vi "Facade.vi"(0 "Data In":T4, 2 "Display State In":T2, 3 "Container State":T3) -> (6 "Data Out":T4, 7 "Display State Out":T2, 8 "Action":T1)   [LabVIEW 2015, in "TTLWaterDelivery.xctl"]
uses:
  TTLWaterDelivery.xctl
  Data.ctl
  Device Classes/WaterDelivery Class/TTLWaterDelivery.lvclass
  <vilib>/_xctls/Container State.ctl
  State.ctl
  <vilib>/_xctls/Action.ctl
  Device Classes/WaterDelivery Class/TTLWaterDelivery.lvclass/TTLWaterDelivery.ctl
  Device Classes/WaterDelivery Class/Read uL_ms.vi
  Device Classes/WaterDelivery Class/Write uL_ms.vi
  <vilib>/_xctls/XControlSupport.lvlib
panel:
  in  "Calibrate":bool
  in  "Sensitivity":dbl format="%#_g ul/ms"
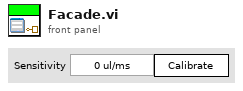
[diagram p1: front panel]
types:
  T1 = typedef "XControlSupport.lvlib/Action.ctl" = cluster{"Data Changed?":bool, "State Changed?":bool, "Action Name":string}
  T2 = typedef "TTLWaterDelivery.xctl/State.ctl" = cluster{"Cal signal":refnum<vi>}
  T3 = typedef "XControlSupport.lvlib/Container State.ctl" = cluster{"Indicator?":bool, "Run Mode?":bool, " Refnum":refnum<vi>}
  T4 = typedef "TTLWaterDelivery.xctl/Data.ctl" = refnum<class "TTLWaterDelivery.lvclass">
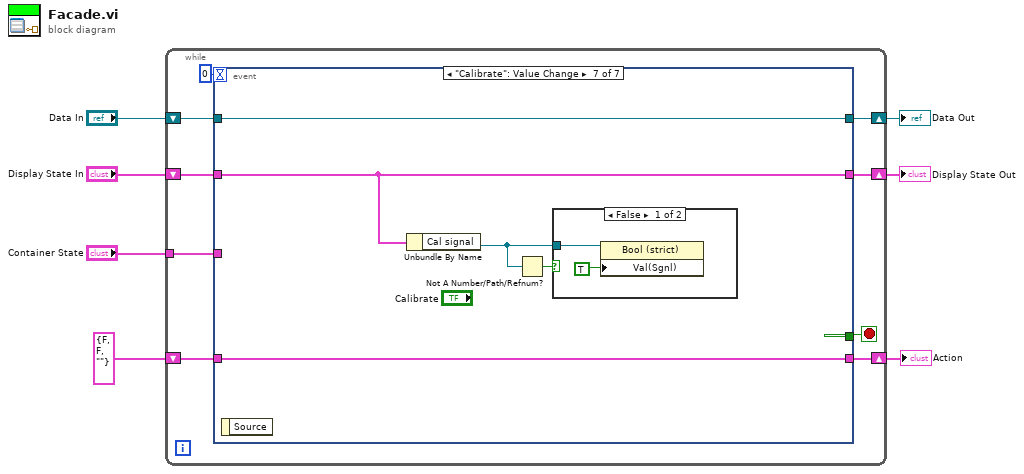
[diagram p0: block diagram]
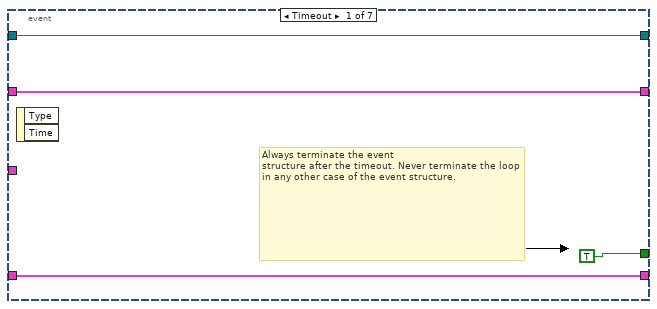
[diagram p2: hidden frame]
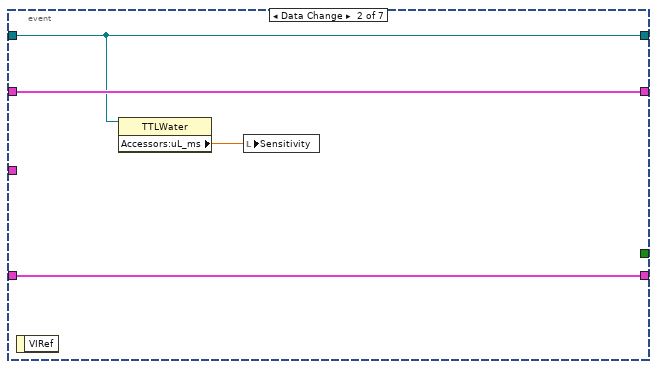
[diagram p3: hidden frame]
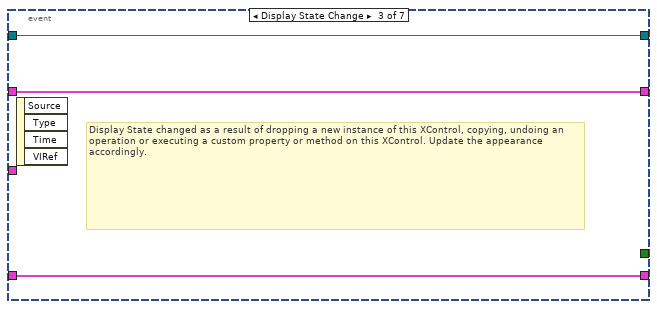
[diagram p4: hidden frame]
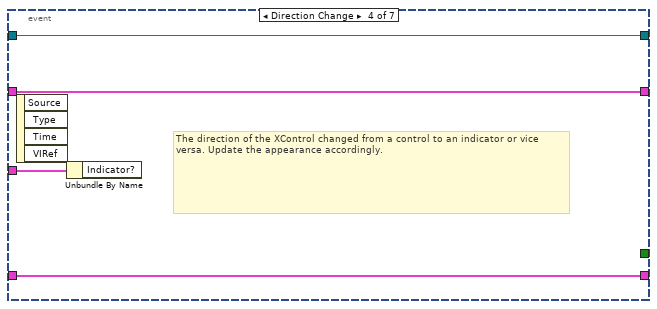
[diagram p5: hidden frame]
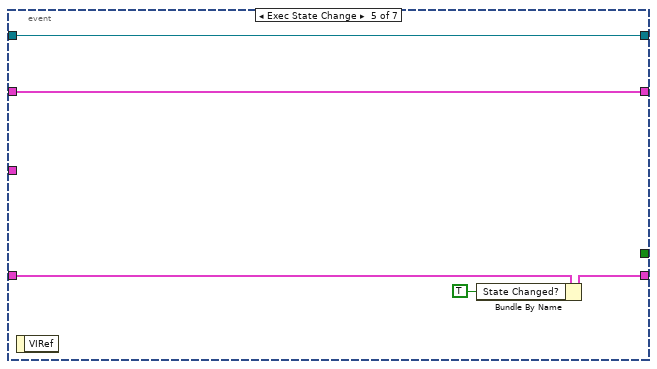
[diagram p6: hidden frame]
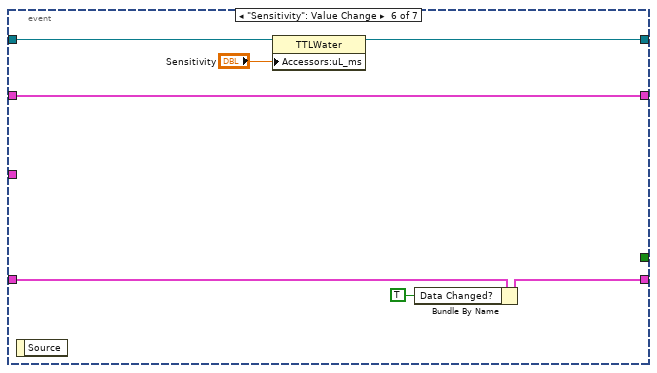
[diagram p7: hidden frame]
diagram:
  n1 = while {
    shift-right: [w15] -> w4
    shift-left: "Display State In" -> [w16]
    tunnel: "Container State" -> [w12]
    shift-right: [w10] -> w7
    shift-left: "Data In" -> [w11]
    shift-right: [w8] -> w2
    shift-left: T1 {"Data Changed?"=FALSE, "State Changed?"=FALSE, "Action Name"=""} ("Action") -> [w9]
    stop <- w14 stop-if-true
    n2 = event shown="[6] \"Calibrate\": Value Change" {
      selector: _ -> [_ _ _ _ _ _ _]
      dyn-events: _ -> [_ _ _ _ _ _ _]
      timeout: 0 -> [_ _ _ _ _ _ _]
      tunnel: w16 -> [w18 w24 w27 w30 w36 w43 w46]
      tunnel: [w18 w24 w27 w30 w36 w43 w46] -> w15
      tunnel: [TRUE _ _ _ _ _ _] -> w14
      tunnel: w12 -> [_ _ _ w31 _ _ _]
      tunnel: w11 -> [w17 w22 w26 w29 w35 w42 w48]
      tunnel: [w17 w22 w26 w29 w35 w40 w48] -> w10
      tunnel: [w19 w23 w25 w28 w33 w38 w47] -> w8
      tunnel: w9 -> [w19 w23 w25 w28 w34 w41 w47]
      event Timeout {
        # "Always terminate the event\nstructure after the timeout. Never terminate the loop in any other case of the event structure."
        n3 = event-data() -> ()  [unwired: 1 in, 2 out]
      }
      event Data Change {
        n4 = event-data() -> ()  [unwired: 1 in, 1 out]
        n5 = property class="TTLWater"(reference=w22) -> ("Accessors:uL_ms"=w21:dbl)  [unwired: 1 in, 2 out]
        n6 = local write "Sensitivity"(w21) -> ()
      }
      event Display State Change {
        # "Display State changed as a result of dropping a new instance of this XControl, copying, undoing an operation or executing a custom property or method on this XControl. Update the appearance accordingly."
        n7 = event-data() -> ()  [unwired: 1 in, 4 out]
      }
      event Direction Change {
        # "The direction of the XControl changed from a control to an indicator or vice versa. Update the appearance accordingly."
        n8 = event-data() -> ()  [unwired: 1 in, 4 out]
        n9 = Unbundle By Name(w31) -> ()  [unwired: 1 out]
      }
      event Exec State Change {
        n10 = event-data() -> ()  [unwired: 1 in, 1 out]
        n11 = Bundle By Name(cluster=w34, "State Changed?"=TRUE) -> (w33:T1)
      }
      event "Sensitivity": Value Change {
        n12 = event-data() -> ()  [unwired: 1 in, 1 out]
        n13 = property class="TTLWater"(reference=w42, "Accessors:uL_ms"="Sensitivity") -> (reference out=w40:T4)  [unwired: 1 in, 1 out]
        n14 = Bundle By Name(cluster=w41, "Data Changed?"=TRUE) -> (w38:T1)
      }
      event "Calibrate": Value Change {
        n15 = event-data() -> ()  [unwired: 1 in, 1 out]
        n16 = Unbundle By Name(w46) -> ("Cal signal"=w45:refnum<vi>)
        n17 = Not A Number/Path/Refnum?(number/path/refnum=w45) -> (NaN/Path/Refnum?=w44:bool)
        n18 = case shown="False" w44 {
          tunnel: w45 -> [w50 _]
          frame False {
            n19 = property class="Bool (strict)"(reference=w50, "Val(Sgnl)"=TRUE) -> ()  [unwired: 1 in, 2 out]
          }
          frame True {
          }
        }
      }
    }
  }
  "Display State Out" <- w4
  "Data Out" <- w7
  "Action" <- w2
